vi "Rearrange images (15..05).vi"(0 "Selet tab":enum16{"Diagnostics", "Main"}(ring), 1 "Image indicator layouts 2":T1(array[cluster])=[{"NumberOfImageIndicators"=0.0, "ImageSpecificData"=[{"Width"=0.0, "Left"=0.0, "Top"=0.0, "Image Percentage"={"Height"=0.0, "Width correction"=0.0, "Height correction"=0.0, "Left correction"=0.0, "Top correction"=0.0}, "String Percentage"={"Height"=0.0, "Width correction"=0.0, "Height correction"=0.0, "Left correction"=0.0, "Top correction"=0.0}}, {"Width"=0.0, "Left"=0.0, "Top"=0.0, "Image Percentage"={"Height"=0.0, "Width correction"=0.0, "Height correction"=0.0, "Left correction"=0.0, "Top correction"=0.0}, "String Percentage"={"Height"=0.0, "Width correction"=0.0, "Height correction"=0.0, "Left correction"=0.0, "Top correction"=0.0}}, {"Width"=0.5, "Left"=0.0, "Top"=0.0, "Image Percentage"={"Height"=0.45, "Width correction"=-10.0, "Height correction"=0.0, "Left correction"=0.0, "Top correction"=0.0}, "String Percentage"={"Height"=0.05, "Width correction"=-5.0, "Height correction"=0.0, "Left correction"=0.0, "Top correction"=0.0}}, {"Width"=0.5, "Left"=0.0, "Top"=0.5, "Image Percentage"={"Height"=0.0, "Width correction"=-10.0, "Height correction"=0.0, "Left correction"=0.0, "Top correction"=0.0}, "String Percentage"={"Height"=0.0, "Width correction"=-5.0, "Height correction"=0.0, "Left correction"=0.0, "Top correction"=0.0}}, {"Width"=0.5, "Left"=0.5, "Top"=0.0, "Image Percentage"={"Height"=0.95, "Width correction"=-10.0, "Height correction"=0.0, "Left correction"=0.0, "Top correction"=0.0}, "String Percentage"={"Height"=0.05, "Width correction"=-5.0, "Height correction"=0.0, "Left correction"=0.0, "Top correction"=0.0}}]}, {"NumberOfImageIndicators"=0.0, "ImageSpecificData"=[]}, {"NumberOfImageIndicators"=0.0, "ImageSpecificData"=[{"Width"=0.5, "Left"=0.0, "Top"=0.0, "Image Percentage"={"Height"=0.45, "Width correction"=-7.0, "Height correction"=0.0, "Left correction"=0.0, "Top correction"=0.0}, "String Percentage"={"Height"=0.05, "Width correction"=-5.0, "Height correction"=0.0, "Left correction"=0.0, "Top correction"=0.0}}, {"Width"=0.5, "Left"=0.0, "Top"=0.5, "Image Percentage"={"Height"=0.45, "Width correction"=-7.0, "Height correction"=0.0, "Left correction"=0.0, "Top correction"=0.0}, "String Percentage"={"Height"=0.05, "Width correction"=-5.0, "Height correction"=0.0, "Left correction"=0.0, "Top correction"=0.0}}, {"Width"=0.5, "Left"=0.5, "Top"=0.0, "Image Percentage"={"Height"=0.95, "Width correction"=-7.0, "Height correction"=0.0, "Left correction"=0.0, "Top correction"=0.0}, "String Percentage"={"Height"=0.05, "Width correction"=-5.0, "Height correction"=0.0, "Left correction"=0.0, "Top correction"=0.0}}, {"Width"=0.5, "Left"=0.0, "Top"=0.5, "Image Percentage"={"Height"=0.45, "Width correction"=-7.0, "Height correction"=0.0, "Left correction"=0.0, "Top correction"=0.0}, "String Percentage"={"Height"=0.05, "Width correction"=-5.0, "Height correction"=0.0, "Left correction"=0.0, "Top correction"=0.0}}, {"Width"=0.5, "Left"=0.5, "Top"=0.0, "Image Percentage"={"Height"=0.0, "Width correction"=-7.0, "Height correction"=0.0, "Left correction"=0.0, "Top correction"=0.0}, "String Percentage"={"Height"=0.0, "Width correction"=-5.0, "Height correction"=0.0, "Left correction"=0.0, "Top correction"=0.0}}]}], 5 "Camera names":string[](array[string]), 7 "Type of label":u16(ring) items=["Combo", "String"], 9 "References":T2, 11 "error in (no error)":errorcluster) -> (15 "error out":errorcluster)   [LabVIEW 2019, in "ZenGage v3.0 UI.lvclass"]
uses:
  ZenGage v3.0 UI.lvclass
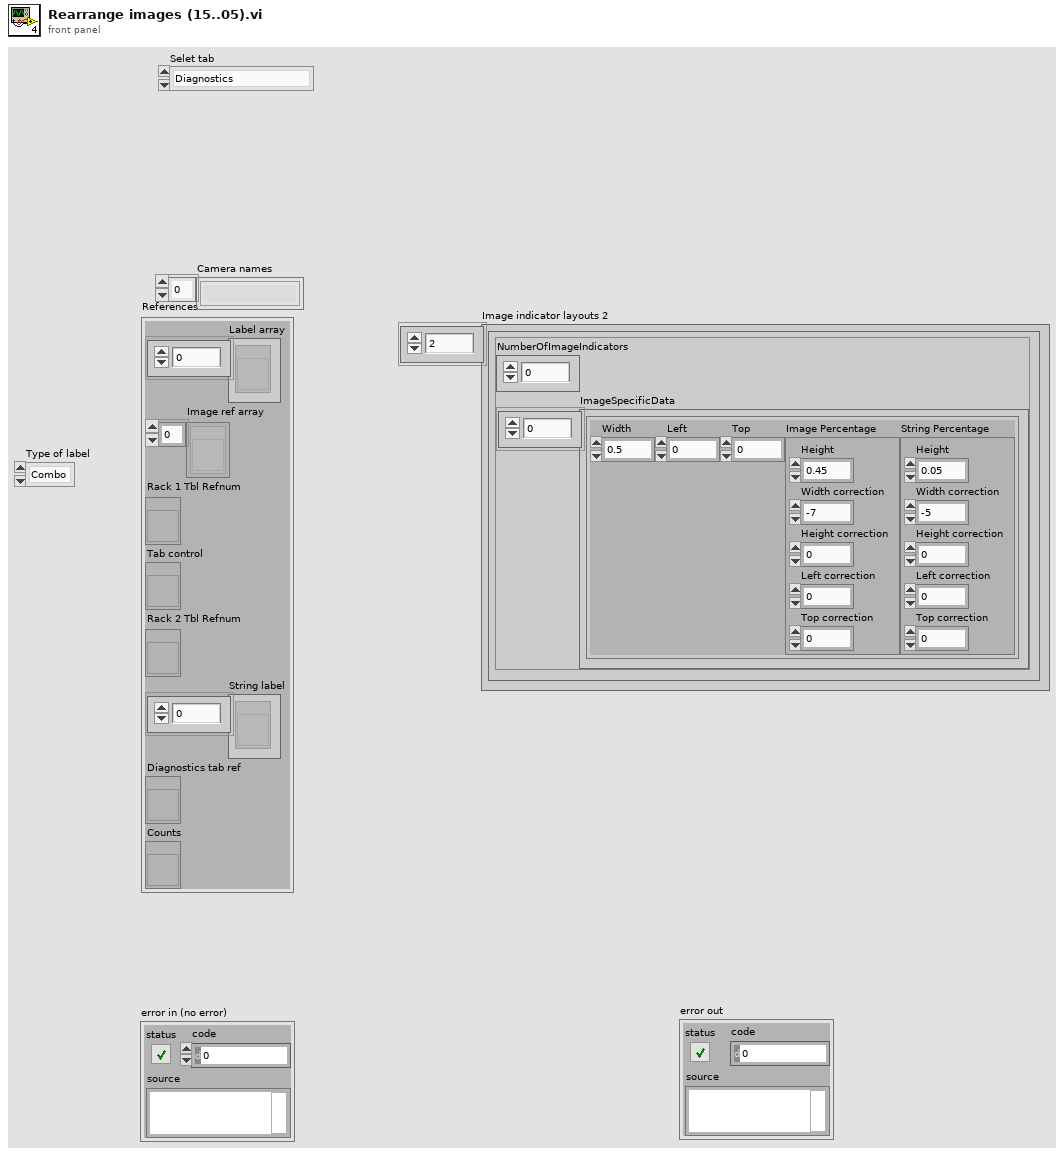
[diagram p1: front panel]
types:
  T1 = cluster{"NumberOfImageIndicators":dbl, "ImageSpecificData":cluster{"Width":dbl, "Left":dbl, "Top":dbl, "Image Percentage":cluster{"Height":dbl, "Width correction":dbl, "Height correction":dbl, "Left correction":dbl, "Top correction":dbl}, "String Percentage":cluster{"Height":dbl, "Width correction":dbl, "Height correction":dbl, "Left correction":dbl, "Top correction":dbl}}[]}[]
  T2 = cluster{"Label array":refnum<vi>[], "Image ref array":refnum<vi>[], "Rack 1 Tbl Refnum":refnum<vi>, "Tab control":refnum<vi>, "Rack 2 Tbl Refnum":refnum<vi>, "String label":refnum<vi>[], "Diagnostics tab ref":refnum<vi>, "Counts":refnum<vi>}
  T3 = cluster{"NumberOfImageIndicators":dbl, "ImageSpecificData":cluster{"Width":dbl, "Left":dbl, "Top":dbl, "Image Percentage":cluster{"Height":dbl, "Width correction":dbl, "Height correction":dbl, "Left correction":dbl, "Top correction":dbl}, "String Percentage":cluster{"Height":dbl, "Width correction":dbl, "Height correction":dbl, "Left correction":dbl, "Top correction":dbl}}[]}
  T4 = cluster{"Width":dbl, "Left":dbl, "Top":dbl, "Image Percentage":cluster{"Height":dbl, "Width correction":dbl, "Height correction":dbl, "Left correction":dbl, "Top correction":dbl}, "String Percentage":cluster{"Height":dbl, "Width correction":dbl, "Height correction":dbl, "Left correction":dbl, "Top correction":dbl}}[]
  T5 = cluster{"Tab width":u32, "Tab height":u32, "Left":i32, "Top":i32}
  T6 = cluster{"Width":dbl, "Left":dbl, "Top":dbl, "Image Percentage":cluster{"Height":dbl, "Width correction":dbl, "Height correction":dbl, "Left correction":dbl, "Top correction":dbl}, "String Percentage":cluster{"Height":dbl, "Width correction":dbl, "Height correction":dbl, "Left correction":dbl, "Top correction":dbl}}
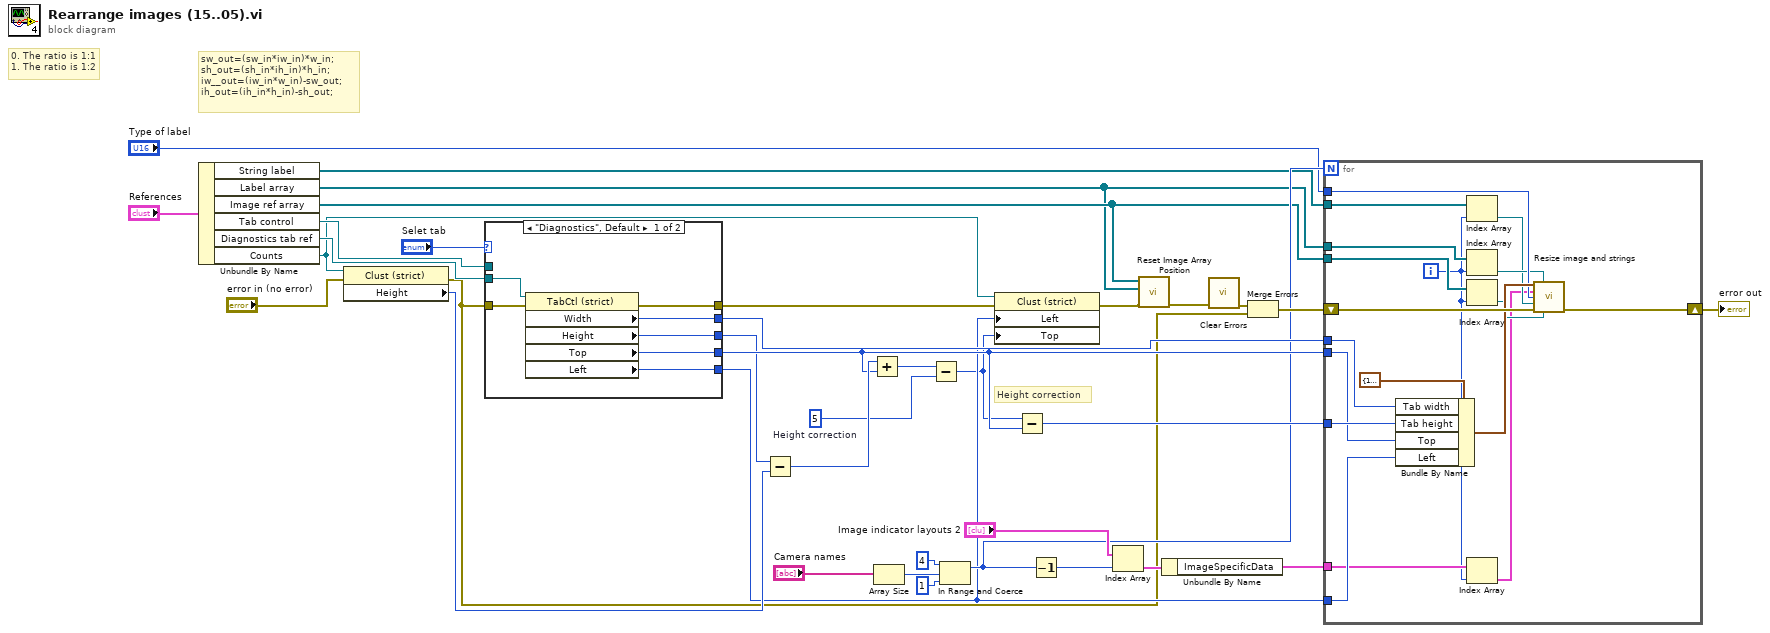
[diagram p0: block diagram]
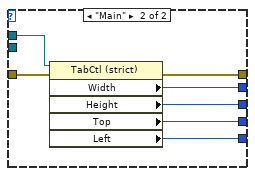
[diagram p2: hidden frame]
diagram:
  w27 = u32 5  # Height correction
  # "Height correction"
  # "sw_out=(sw_in*iw_in)*w_in;\nsh_out=(sh_in*ih_in)*h_in;\niw__out=(iw_in*w_in)-sw_out;\nih_out=(ih_in*h_in)-sh_out;"
  # "0. The ratio is 1:1\n1. The ratio is 1:2"
  n1 = Unbundle By Name("References") -> ("String label"=w10:refnum<vi>[], "Label array"=w1:refnum<vi>[], "Image ref array"=w3:refnum<vi>[], "Tab control"=w29:refnum<vi>, "Diagnostics tab ref"=w7:refnum<vi>, "Counts"=w6:refnum<vi>)
  n2 = property on="Property Node" class="Clust (strict)"(reference=w6, error in="error in (no error)") -> (error out=w2:errorcluster, "Height"=w34:u32)  [unwired: 1 out]
  n3 = case shown="\"Diagnostics\", Default" "Selet tab" {
    tunnel: [w39 w50] -> w31
    tunnel: w29 -> [_ w49]
    tunnel: [w40 w48] -> w28
    tunnel: [w41 w47] -> w26
    tunnel: [w42 w46] -> w22
    tunnel: w2 -> [w43 w45]
    tunnel: [w38 w44] -> w13
    tunnel: w7 -> [w37 _]
    frame "Diagnostics", Default {
      n4 = property class="TabCtl (strict)"(reference=w37, error in=w43) -> (error out=w42:errorcluster, "Width"=w41:u32, "Height"=w40:u32, "Top"=w39:i32, "Left"=w38:i32)  [unwired: 1 out]
    }
    frame "Main" {
      n5 = property class="TabCtl (strict)"(reference=w49, error in=w45) -> (error out=w46:errorcluster, "Width"=w47:u32, "Height"=w48:u32, "Top"=w50:i32, "Left"=w44:i32)  [unwired: 1 out]
    }
  }
  n6 = Subtract(x=w28, y=w34) -> (x-y=w36:u32)
  n7 = Add(x=w36, y=w31) -> (x+y=w35:u32)
  n8 = Array Size(array="Camera names") -> (size(s)=w16:i32)
  n9 = Subtract(x=w35, y=w27) -> (x-y=w12:u32)
  n10 = In Range and Coerce(upper limit=4 ("size(s)"), x=w16, lower limit=1 ("size(s)")) -> (coerced(x)=w15:i32)  [unwired: 1 out]
  n11 = property on="Property Node" class="Clust (strict)"(reference=w6, error in=w22, "Left"=w13, "Top"=w12) -> (error out=w5:errorcluster)  [unwired: 1 out]
  n12 = Subtract(x=w12, y=w31) -> (x-y=w33:u32)
  n13 = Decrement(x=w15) -> (x-1=w20:i32)
  n14 = Index Array(array="Image indicator layouts 2", index=w20) -> (element=w24:T3)
  n15 = call "Reset Image Array Position.vi"("error in (no error)"=w5, "Label array"=w1, "Image ref array"=w3) -> ("error in (no error)"=w4:errorcluster)  [unwired: 8 in]
  n16 = Unbundle By Name(w24) -> ("ImageSpecificData"=w23:T4)
  n17 = call <vilib>:"Clear Errors.vi"("error in (no error)"=w4) -> ("error out"=w11:errorcluster)  [unwired: 5 in, 1 out]
  n18 = Merge Errors(w11, w2) -> (w21:errorcluster)
  n19 = for {
    N: w15 -> [_]
    tunnel: w33 -> [w65]
    tunnel: w26 -> [w66]
    tunnel: w1 -> [w59]
    tunnel: w3 -> [w58]
    tunnel: w23 -> [w53]
    shift-right: [w67] -> w32
    shift-left: w21 -> [w68]
    tunnel: w13 -> [w61]
    tunnel: w31 -> [w62]
    tunnel: "Type of label" -> [w60]
    tunnel: w10 -> [w57]
    i -> [w51]
    n20 = Bundle By Name(cluster=T5 {"Tab width"=1176, "Tab height"=619, "Left"=0, "Top"=0} ("Tab details"), "Tab width"=w66, "Tab height"=w65, "Top"=w62, "Left"=w61) -> (w63:T5)
    n21 = Index Array(array=w57, index=w51) -> (element=w55:refnum<vi>)
    n22 = Index Array(array=w59, index=w51) -> (element=w56:refnum<vi>)
    n23 = Index Array(array=w58, index=w51) -> (element=w54:refnum<vi>)
    n24 = Index Array(array=w53, index=w51) -> (element=w52:T6)
    n25 = call "Resize image and strings.vi"("Tab details"=w63, "Image label"=w56, "Image position and resize"=w52, "Type of label"=w60, "TL"=w55, "error in (no error)"=w68, "Img Refnum"=w54) -> ("error out"=w67:errorcluster)  [unwired: 8 in]
  }
  "error out" <- w32
